vi "SFCS_GetMAC_ByUSNITEM.vi"() -> (0 "Status (NG or MAC address)":string)   [LabVIEW 2011]
uses:
  Instance           3 29Saved   SFCS_GetMAC_ByUSNITEM .vi
  Instance           8 29Saved   SFCS_GetMAC_ByUSNITEM .vi
  Instance           9 29Saved   SFCS_GetMAC_ByUSNITEM .vi
  Instance          10 29Saved   SFCS_GetMAC_ByUSNITEM .vi
  Instance          13 29Saved   SFCS_GetMAC_ByUSNITEM .vi
  Instance          17 29Saved   SFCS_GetMAC_ByUSNITEM .vi
panel:
  out "軟體版本 Software Version":string
  out "begin time":u32
  out "SN":string
  out "Category":string
  out "STAGE":string
  out "SFCS_IP":string
  out "Status":bool
  in  "URL":string
  # "Get MAC (SFCS_USNItem)"
  # "2014-12-15"
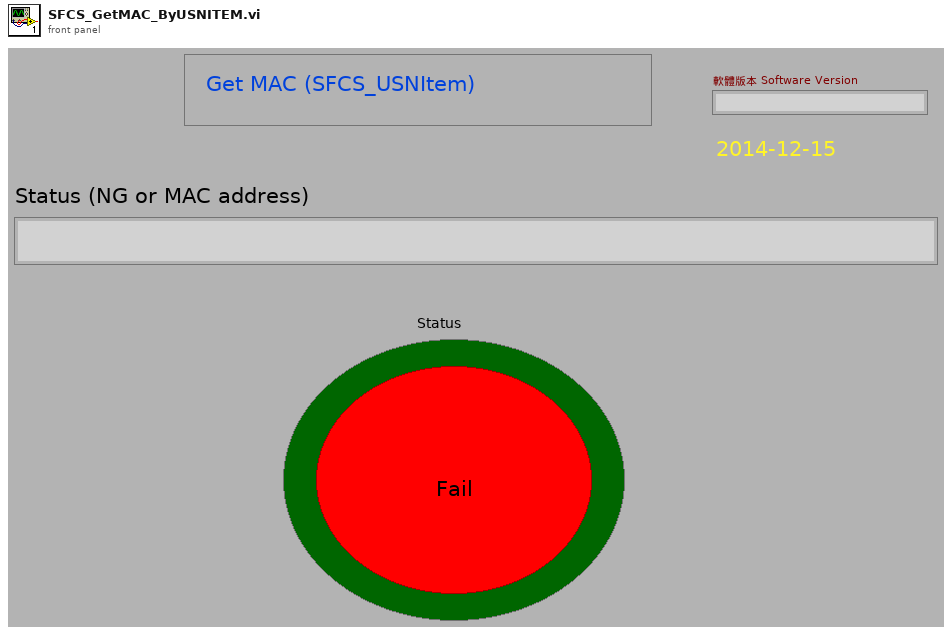
[diagram p1: front panel]
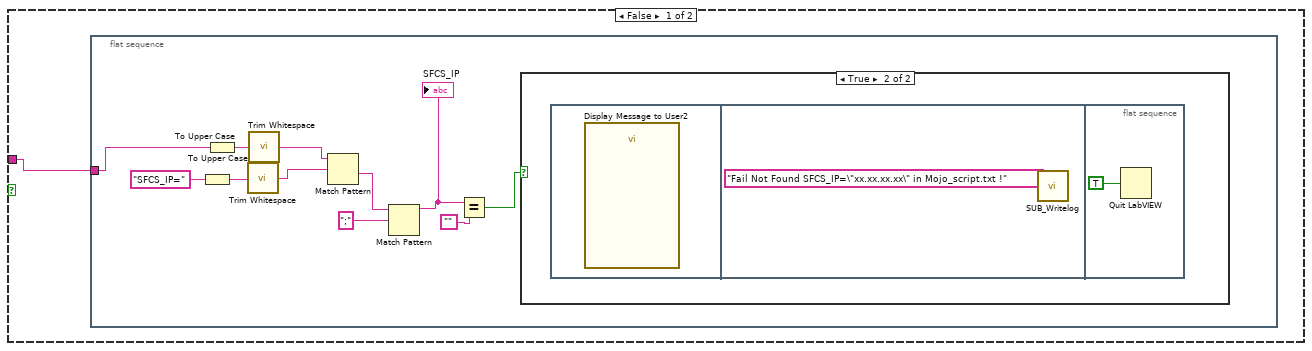
[diagram p4: hidden frame]
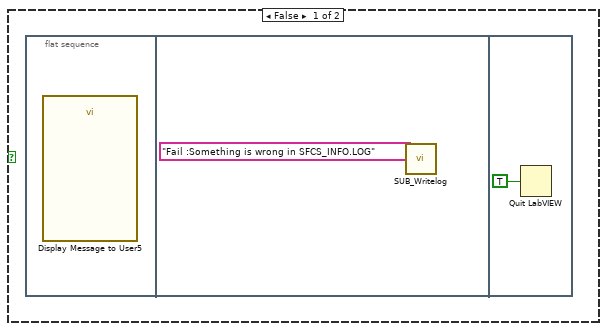
[diagram p7: hidden frame]
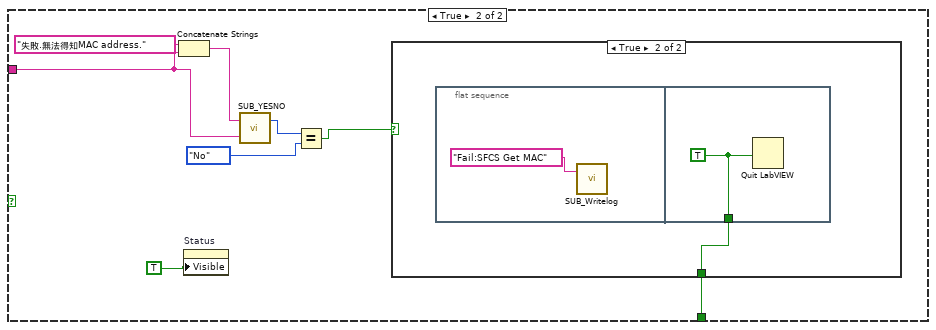
[diagram p9: hidden frame]
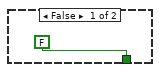
[diagram p10: hidden frame]
diagram:
  n1 = flat-sequence {
    tunnel: [w12] -> w1
    tunnel: w1 -> [w33]
    frame #0 {
      n2 = Tick Count (ms)() -> (millisecond timer value=→"begin time":u32)
    }
    frame #1 {
      n3 = property on="Status" class="Bool (strict)"("Visible"=FALSE) -> ()  [unwired: 2 in, 2 out]
    }
    frame #2 {
      n4 = call "SUB_SW_Version.vi"() -> ("Current Software Version"=→"軟體版本 Software Version":string)  [unwired: 3 in]
    }
    frame #3 {
      n5 = case shown="True" TRUE {
        frame False {
        }
        frame True {
          n6 = call "SUB_SearchFile_inFolder.vi"("Search Filename in Folder"="SFCS_INFO.LOG") -> ("File Existing True/Flase"=w6:bool)  [unwired: 1 in]
          n7 = case shown="False" w6 {
            frame False {
              n8 = flat-sequence {
                frame #0 {
                  n9 = call "Display Message to User3"() -> ()  [unwired: 10 in, 2 out]
                }
                frame #1 {
                  n10 = call "SUB_Writelog.vi"("Pass/Fail"="Fail :Please Do Check Route First !") -> ()  [unwired: 2 in]
                }
                frame #2 {
                  n11 = Quit LabVIEW(quit? (T)=TRUE) -> ()
                }
              }
            }
            frame True {
            }
          }
        }
      }
    }
    frame #4 {
      n12 = call "SUB_DELETE_SpecificFile.vi"("Filename to be  Deleted"="PQAW_MAC.log") -> ()  [unwired: 2 in, 1 out]
    }
    frame #5 {
      n13 = call "SUB_Read_specifFile.vi"("name or relative path"="S8300E_sfcs_misc.TXT" ("Script FileName")) -> ("error out"=w15:errorcluster, "text"=w12:string)  [unwired: 1 in]
      n14 = Unbundle By Name(w15) -> ("code"=w14:i32)
      n15 = Not Equal To 0?(x=w14) -> (x != 0?=w13:bool)
      n16 = case shown="True" w13 {
        tunnel: w12 -> [w16 _]
        frame False {
          n17 = flat-sequence {
            tunnel: w16 -> [w22]
            frame #0 {
              n18 = To Upper Case(1:"SFCS_IP=" ("string")) -> (0:w26:string)
              n19 = To Upper Case(1:w22) -> (0:w27:string)
              n20 = call <vilib>:"Trim Whitespace.vi"("string"=w26) -> ("trimmed string"=w24:string)  [unwired: 1 in]
              n21 = call <vilib>:"Trim Whitespace.vi"("string"=w27) -> ("trimmed string"=w23:string)  [unwired: 1 in]
              n22 = Match Pattern(string=w23, regular expression=w24) -> (after substring=w21:string)  [unwired: 1 in, 3 out]
              n23 = Match Pattern(string=w21, regular expression=";") -> (before substring=w19:string)  [unwired: 1 in, 3 out]
              "SFCS_IP" <- w19
              n24 = Equal?(x=w19, y="") -> (x = y?=w17:bool)
              n25 = case shown="True" w17 {
                frame False {
                }
                frame True {
                  n26 = flat-sequence {
                    frame #0 {
                      n27 = call "Display Message to User2"() -> ()  [unwired: 10 in, 2 out]
                    }
                    frame #1 {
                      n28 = call "SUB_Writelog.vi"("Pass/Fail"="Fail Not Found SFCS_IP=\"xx.xx.xx.xx\" in Mojo_script.txt !") -> ()  [unwired: 2 in]
                    }
                    frame #2 {
                      n29 = Quit LabVIEW(quit? (T)=TRUE) -> ()
                    }
                  }
                }
              }
            }
          }
        }
        frame True {
          n30 = flat-sequence {
            frame #0 {
              n31 = call "Display Message to User"() -> ()  [unwired: 10 in, 2 out]
            }
            frame #1 {
              n32 = call "SUB_Writelog.vi"("Pass/Fail"="Fail Mojo_script.txt is Missing!") -> ()  [unwired: 2 in]
            }
            frame #2 {
              n33 = Quit LabVIEW(quit? (T)=TRUE) -> ()
            }
          }
        }
      }
    }
    frame #6 {
      n34 = To Upper Case(1:"SFCS_STAGE=" ("string")) -> (0:w54:string)
      n35 = To Upper Case(1:w33) -> (0:w55:string)
      n36 = To Upper Case(1:"SFCS_MAC_Category=" ("string")) -> (0:w47:string)
      n37 = To Upper Case(1:w33) -> (0:w48:string)
      n38 = call <vilib>:"Trim Whitespace.vi"("string"=w54) -> ("trimmed string"=w53:string)  [unwired: 1 in]
      n39 = call <vilib>:"Trim Whitespace.vi"("string"=w55) -> ("trimmed string"=w52:string)  [unwired: 1 in]
      n40 = call <vilib>:"Trim Whitespace.vi"("string"=w47) -> ("trimmed string"=w46:string)  [unwired: 1 in]
      n41 = call <vilib>:"Trim Whitespace.vi"("string"=w48) -> ("trimmed string"=w45:string)  [unwired: 1 in]
      n42 = Match Pattern(string=w52, regular expression=w53) -> (after substring=w51:string)  [unwired: 1 in, 3 out]
      n43 = Match Pattern(string=w45, regular expression=w46) -> (after substring=w44:string)  [unwired: 1 in, 3 out]
      n44 = Match Pattern(string=w51, regular expression=";") -> (before substring=w41:string)  [unwired: 1 in, 3 out]
      "STAGE" <- w41
      n45 = Match Pattern(string=w44, regular expression=";") -> (before substring=w40:string)  [unwired: 1 in, 3 out]
      "Category" <- w40
      n46 = Not Equal?(x=w40, y="") -> (x != y?=w36:bool)
      n47 = Not Equal?(x=w41, y="") -> (x != y?=w37:bool)
      n48 = And(x=w37, y=w36) -> (x .and. y?=w35:bool)
      n49 = And(x=w35, y=TRUE) -> (x .and. y?=w34:bool)
      n50 = case shown="False" w34 {
        frame False {
          n51 = flat-sequence {
            frame #0 {
              n52 = call "Display Message to User4"() -> ()  [unwired: 10 in, 2 out]
            }
            frame #1 {
              n53 = call "SUB_Writelog.vi"("Pass/Fail"="Fail :Stage,Category,Sequence not define in script file!") -> ()  [unwired: 2 in]
            }
            frame #2 {
              n54 = Quit LabVIEW(quit? (T)=TRUE) -> ()
            }
          }
        }
        frame True {
        }
      }
    }
    frame #7 {
      n55 = call "SUB_Read_specifFile.vi"("name or relative path"="SFCS_INFO.LOG") -> ("error out"=w68:errorcluster, "text"=w67:string)  [unwired: 1 in]
      n56 = Unbundle By Name(w68) -> ("code"=w65:i32)
      n57 = call "SUB_FindSpecificString.vi"("Find this String"="USN=", "String data"=w67) -> ("before \"; \" string"=→"SN":string, "Found"=w63:bool)  [unwired: 2 in]
      n58 = Equal?(x=w65, y=0) -> (x = y?=w60:bool)
      n59 = Equal?(x=w63, y=TRUE) -> (x = y?=w61:bool)
      n60 = And(x=w61, y=w60) -> (x .and. y?=w58:bool)
      n61 = case shown="True" w58 {
        frame False {
          n62 = flat-sequence {
            frame #0 {
              n63 = call "Display Message to User5"() -> ()  [unwired: 10 in, 2 out]
            }
            frame #1 {
              n64 = call "SUB_Writelog.vi"("Pass/Fail"="Fail :Something is wrong in SFCS_INFO.LOG") -> ()  [unwired: 2 in]
            }
            frame #2 {
              n65 = Quit LabVIEW(quit? (T)=TRUE) -> ()
            }
          }
        }
        frame True {
        }
      }
    }
    frame #8 {
      n66 = local write "Status"(FALSE ("Status")) -> ()
    }
    frame #9 {
      n67 = local read "SFCS_IP"() -> (w73:string)
      n68 = local write "URL"(w73) -> ()
      n69 = local write "Status (NG or MAC address)"("") -> ()
    }
    frame #10 {
      n70 = while {
        stop <- w86 stop-if-true
        n71 = local read "STAGE"() -> (w78:string)
        n72 = local read "Category"() -> (w75:string)
        n73 = local read "SN"() -> (w79:string)
        n74 = call "SUB_SFCS_GetUSNItem.vi"("URL"="URL", "SN"=w79, "Stage"=w78, "CATEGORY"=w75, "SEQ"=0) -> ("Status"=w77:string)
        "Status (NG or MAC address)" <- w77
        n75 = To Upper Case(1:"NG" ("string")) -> (0:w94:string)
        n76 = To Upper Case(1:w77) -> (0:w95:string)
        n77 = call <vilib>:"Trim Whitespace.vi"("string"=w94) -> ("trimmed string"=w91:string)  [unwired: 1 in]
        n78 = call <vilib>:"Trim Whitespace.vi"("string"=w95) -> ("trimmed string"=w90:string)  [unwired: 1 in]
        n79 = String Length(string=w90) -> (length=w83:i32)
        n80 = Match Pattern(string=w90, regular expression=w91) -> (match substring=w92:string)  [unwired: 1 in, 3 out]
        n81 = Not Equal?(x=w83, y=12) -> (x != y?=w82:bool)
        n82 = Not Equal?(x=w83, y=17) -> (x != y?=w81:bool)
        n83 = Equal?(x=w92, y=w91) -> (x = y?=w88:bool)
        n84 = Not Exclusive Or(1:w81, 2:w82) -> (0:w85:bool)
        n85 = Or(x=w85, y=w88) -> (x .or. y?=w87:bool)
        n86 = case shown="False" w87 {
          tunnel: w77 -> [w96 w132]
          tunnel: [w104 w131] -> w86
          frame False {
            n87 = call "SUB_OUT_THIS_token.vi"("Remove token symbl1 3"=".", "Remove token symbl1 2"=":", "Remove token symbl1"=".", "input string"=w96) -> ("result string"=w102:string)  [unwired: 1 in]
            n88 = flat-sequence {
              tunnel: w102 -> [w106]
              tunnel: [w106] -> w101
              tunnel: [w105] -> w97
              tunnel: w96 -> [w105]
              tunnel: [w116] -> w103
              tunnel: w101 -> [w110]
              tunnel: w97 -> [w109]
              tunnel: w103 -> [w121]
              tunnel: [w130] -> w104
              frame #0 {
                n89 = local write "Status"(TRUE ("Status")) -> ()
                n90 = property on="Status" class="Bool (strict)"("Visible"=TRUE) -> ()  [unwired: 2 in, 2 out]
              }
              frame #1 {
                n91 = call <vilib>:"Trim Whitespace.vi"("string"=w110) -> ("trimmed string"=w115:string)  [unwired: 1 in]
                n92 = To Upper Case(1:w115) -> (0:w112:string)
                n93 = Concatenate Strings("Get  MAC from system=", w109) -> (w116:string)
                n94 = Concatenate Strings("LAN_MAC=", w112, ";") -> (w114:string)
                n95 = call "SUB_WriteMAC_toFile.vi"("MAC Address"=w114) -> ()  [unwired: 2 in]
              }
              frame #2 {
                w120 = "\n"
                n96 = local read "begin time"() -> (w125:u32)
                n97 = Tick Count (ms)() -> (millisecond timer value=w124:u32)
                n98 = call "SUB_CAL_TESTTIME.vi"("Test Item name"="SFCS_GetMAC", "Stop tick time"=w124, "Start tick time"=w125) -> ("Test Time output"=w119:string)  [unwired: 2 in]
                n99 = Concatenate Strings("Pass : SFCS_GETMAC" ("Pass/Fail"), w120, w121, w120, w119) -> (w118:string)
                n100 = call "SUB_Writelog.vi"("Pass/Fail"=w118) -> ()  [unwired: 2 in]
              }
              frame #3 {
                n101 = case shown="True" FALSE {
                  frame False {
                  }
                  frame True {
                    n102 = local read "Status (NG or MAC address)"() -> (w128:string)
                    n103 = Concatenate Strings("從系統的訊息" ("string"), w128) -> (w127:string)
                    n104 = call "Display Message to User6"("Message"=w127) -> ()  [unwired: 9 in, 2 out]
                  }
                }
              }
              frame #4 {
                w130 = TRUE ("quit? (T)")
                n105 = Quit LabVIEW(quit? (T)=w130) -> ()
              }
            }
          }
          frame True {
            n106 = Concatenate Strings("失敗.無法得知MAC address." ("string"), w132) -> (w133:string)
            n107 = property on="Status" class="Bool (strict)"("Visible"=TRUE) -> ()  [unwired: 2 in, 2 out]
            n108 = call "SUB_YESNO.vi"("Debug View"=w132, "Status"=w133) -> ("yes/no"=w138:enum32{"No Selection", "Yes", "No", "None"})  [unwired: 1 in]
            n109 = Equal?(x=w138, y=enum32{"No Selection", "Yes", "No", "None"}."No") -> (x = y?=w136:bool)
            n110 = case shown="True" w136 {
              tunnel: [FALSE w140] -> w131
              frame False {
              }
              frame True {
                n111 = flat-sequence {
                  tunnel: [w142] -> w140
                  frame #0 {
                    n112 = call "SUB_Writelog.vi"("Pass/Fail"="Fail:SFCS Get MAC") -> ()  [unwired: 2 in]
                  }
                  frame #1 {
                    w142 = TRUE
                    n113 = Quit LabVIEW(quit? (T)=w142) -> ()
                  }
                }
              }
            }
          }
        }
      }
    }
  }
